vi "Sample-1.vi"() -> ()   [LabVIEW 2016]
uses:
  <vilib>/NI/Modbus Library/API/Modbus API.lvclass/Modbus API.ctl
  <vilib>/NI/Modbus Library/Transmission Data Unit/Transmission Data Unit.lvclass/Transmission Data Unit.ctl
  <vilib>/NI/Modbus Library/Transmission Data Unit/Write Unit ID.vi
  <vilib>/NI/Modbus Library/API/Read Transmission Data Unit.vi
  <vilib>/NI/Modbus Library/API/Write Transmission Data Unit.vi
  <vilib>/NI/Modbus Library/API/Master/Modbus Master.lvclass
  C:/Program Files/National Instruments/LabVIEW 2016/vi.lib/NI/Modbus Library/API/Modbus API.lvclass
  <vilib>/NI/Modbus Library/API/Wrapper/Create TCP Master.vi
  <vilib>/NI/Modbus Library/API/Wrapper/API Main.lvlib
panel:
  in  "stop":bool
  out "Tab Control":T1(tab)
  out "PM-01-FREQ":dbl
  out "PM-01-IAC":dbl
  out "PM-01-VAC":dbl
  out "PM-01-PAC":dbl
  out "SI-01-FREQ":dbl
  out "SI-01-L3":dbl
  out "SI-01-L2":dbl
  out "SI-01-L1":dbl
  out "SI-01-PAC":dbl
  out "SB-02-B-IAC":dbl
  out "SB-02-B-VAC":dbl
  out "SB-02-A-IAC":dbl
  out "SB-02-A-VAC":dbl
  out "SB-02-PAC":dbl
  out "SI-M-FREQ":dbl
  out "SI-M-L3":dbl
  out "SI-M-L2":dbl
  out "SI-M-L1":dbl
  out "SI-M-PAC":dbl
  out "BANK-02-TEMP":dbl
  out "BANK-02-IDC":dbl
  out "BANK-02-VDC":dbl
  out "BANK-02-SOC":dbl
  out "BANK-01-TEMP":dbl
  out "BANK-01-IDC":dbl
  out "BANK-01-VDC":dbl
  out "BANK-01-SOC":dbl
  out "SB-01-B-IAC":dbl
  out "SB-01-B-VAC":dbl
  out "SB-01-A-IAC":dbl
  out "SB-01-A-VAC":dbl
  out "SB-01-PAC":dbl
  in  "Interval":string(combo)
  in  "setting_save_mysql":bool
  in  "db_pwd":string caption="SB-01-IPADDRESS"
  in  "db_username":string caption="SB-01-IPADDRESS"
  in  "db_database":string caption="SB-01-IPADDRESS"
  in  "db_port":string caption="SB-01-IPADDRESS"
  in  "db_host":string caption="SB-01-IPADDRESS"
  in  "db_connection":string caption="SB-01-IPADDRESS"
  in  "setting_save":bool
  in  "SB-04-PORT":string
  in  "SB-04-IPADDRESS":string caption="SB-01-IPADDRESS"
  in  "SB-03-PORT":string
  in  "SB-03-IPADDRESS":string caption="SB-01-IPADDRESS"
  in  "SB-02-PORT":string
  in  "SB-02-IPADDRESS":string caption="SB-01-IPADDRESS"
  in  "SB-01-PORT":string
  in  "SB-01-IPADDRESS":string
  in  "SB-05-IPADDRESS":string caption="SB-01-IPADDRESS"
  in  "SB-05-PORT":string
  in  "Multicolumn Listbox":i32(listbox)
  in  "Path":path
  in  "DATE_END":timestamp format="%<%d/%m/%Y>T"
  in  "DATE_START":timestamp format="%<%d/%m/%Y>T"
  in  "DOWNLOAD":bool
  out "AC_VOLTAGE":cluster{dbl, dbl}[](graph)
  out "BATTERY_CURRENT":cluster{dbl, dbl}[](graph)
  out "SOC":cluster{dbl, dbl}[](graph)
  out "AC_POWER":cluster{dbl, dbl}[](graph)
  in  "Radio Buttons":T2(radio)
  # "RUMAH KUNJAN ( 8.19 kWp )"
  # "SB-01"
  # "BANK-2"
  # "BANK-1"
  # "SB-02"
  # "SOC (%)"
  # "SOC (%)"
  # "Pac (W)"
  # "Pac (W)"
  # "V_bat(V)"
  # "V_bat(V)"
  # "A.Vdc(V)"
  # "A.Vdc(V)"
  # "I_bat(A)"
  # "I_bat(A)"
  # "A.Idc(A)"
  # "A.Idc(A)"
  # "T_bat(°C)"
  # "T_bat(°C)"
  # "B.Vdc(V)"
  # "B.Vdc(V)"
  # "B.Idc(A)"
  # "B.Idc(A)"
  # "SI-M"
  # "SI-01"
  # "Pac (W)"
  # "Pac (W)"
  # "L1"
  # "L1"
  # "L2"
  # "L2"
  # "L3"
  # "L3"
  # "FREQ(HZ)"
  # "FREQ(HZ)"
  # "PM-01"
  # "Pac(W)"
  # "Vac (V)"
  # "Iac(A)"
  # "Freq(Hz)"
  # "SETTING"
  # "MODBUS TCP IP"
  # "MYSQL DATABASE"
  # "SB-01"
  # "DB_CONNECTION :"
  # "IP ADDRESS"
  # "DB_HOST :"
  # "PORT"
  # "DB_PORT  :"
  # "SB-02"
  # "DB_DATABASE  :"
  # "IP ADDRESS"
  # "DB_USERNAME  :"
  # "PORT"
  # "DB_PASSWORD  :"
  # "INTERVAL  :"
  # "SI-M"
  # "IP ADDRESS"
  # "PORT"
  # "SI-01"
  # "IP ADDRESS"
  # "PORT"
  # "DATA MANAGER"
  # "IP ADDRESS"
  # "PORT"
  # "ALERT LIST"
  # "DOWNLOAD DATA"
  # "FILE"
  # "DATE (START)"
  # "DATE (END)"
  # "CHART"
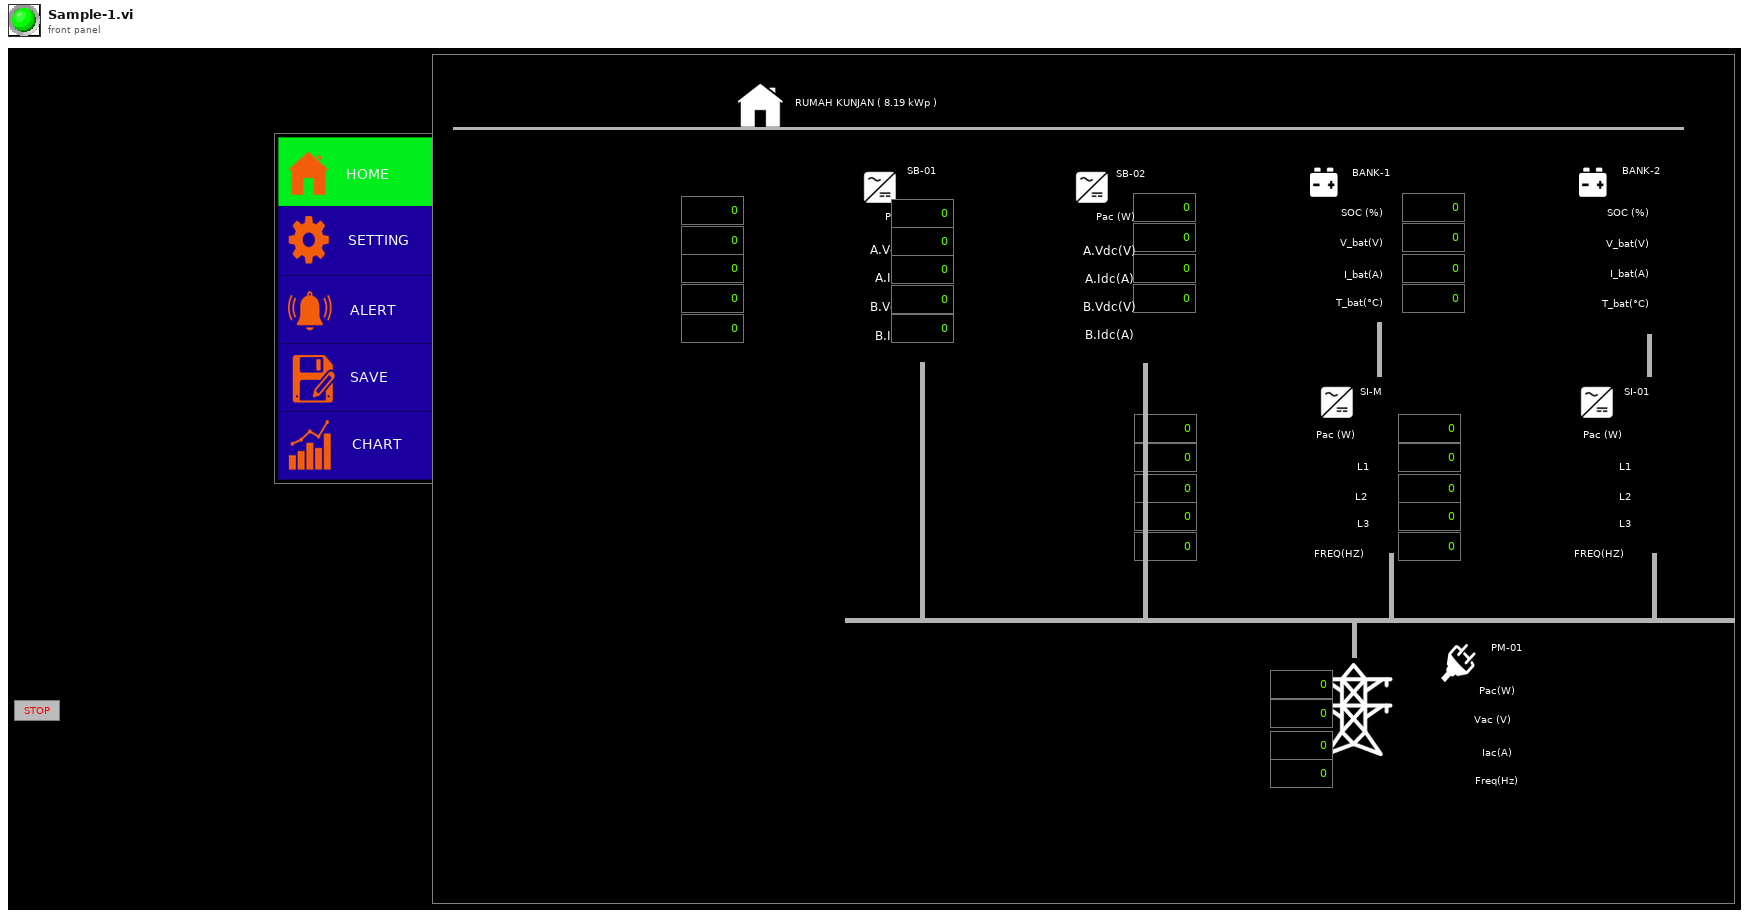
[diagram p1: front panel]
types:
  T1 = enum32{"Page 1", "Page 2", "Page 3", "Page 4", "Page 5"}
  T2 = enum32{"HOME", "SETTING", "ALERT", "SAVE", "CHART"}
  T3 = enum16{"open", "replace", "create", "open or create", "replace or create", "replace or create with confirmation"}
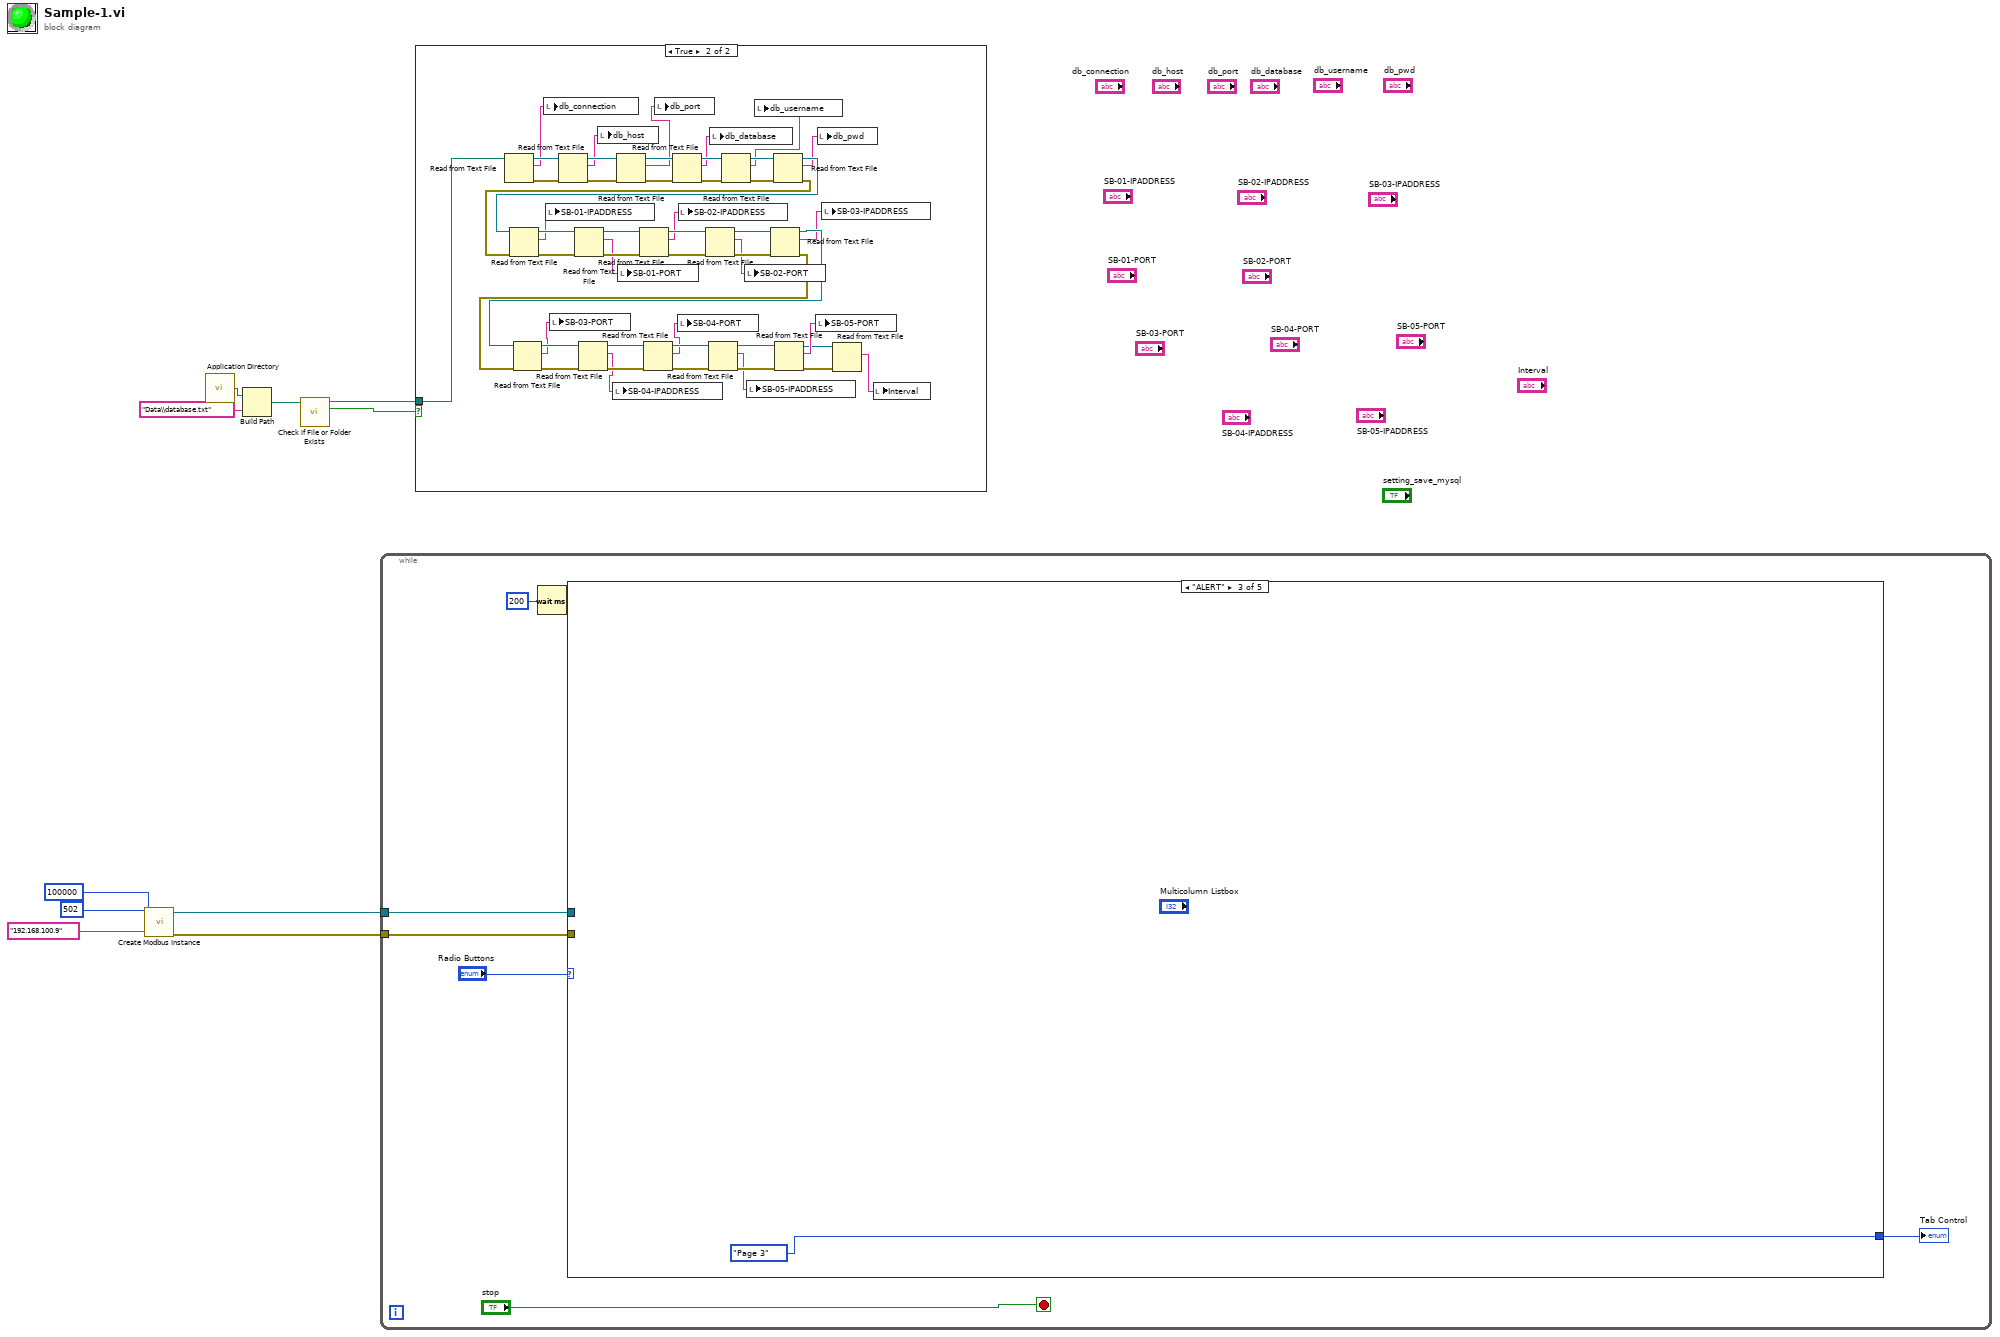
[diagram p0: block diagram]
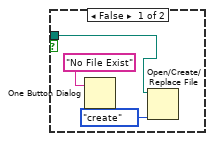
[diagram p2: hidden frame]
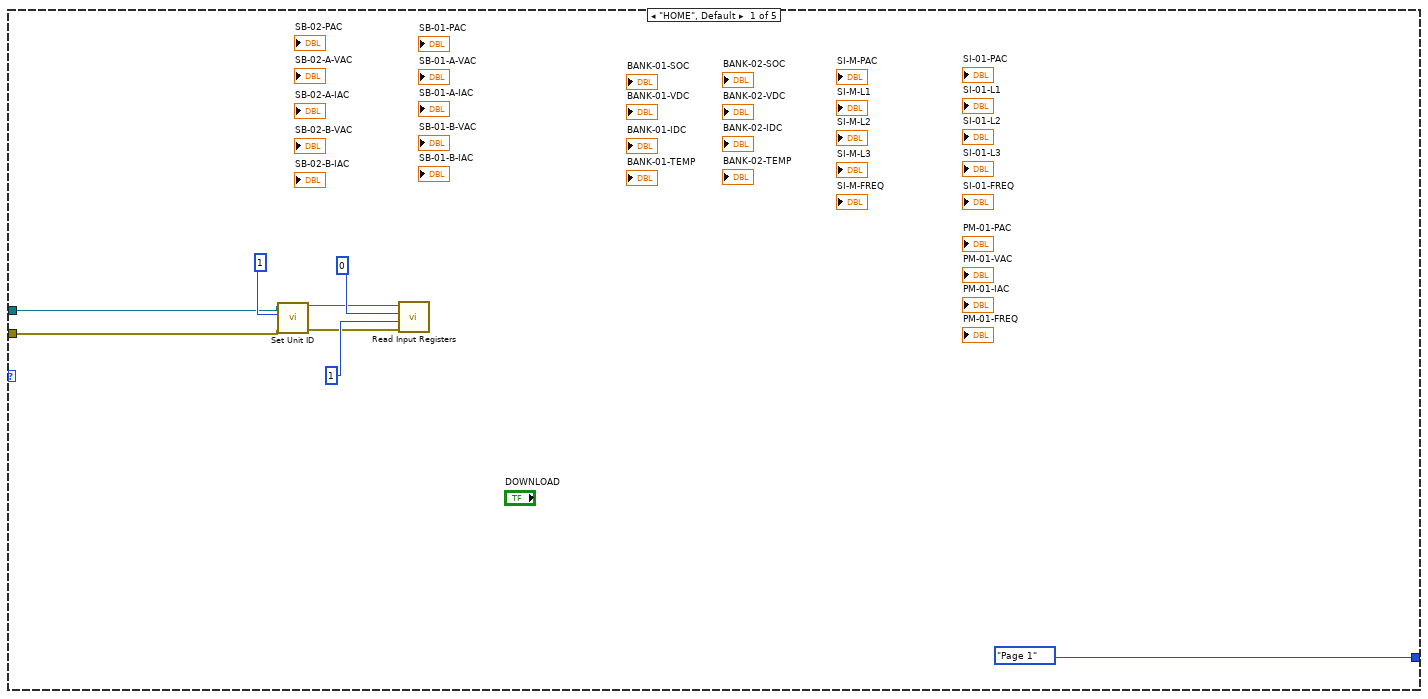
[diagram p3: hidden frame]
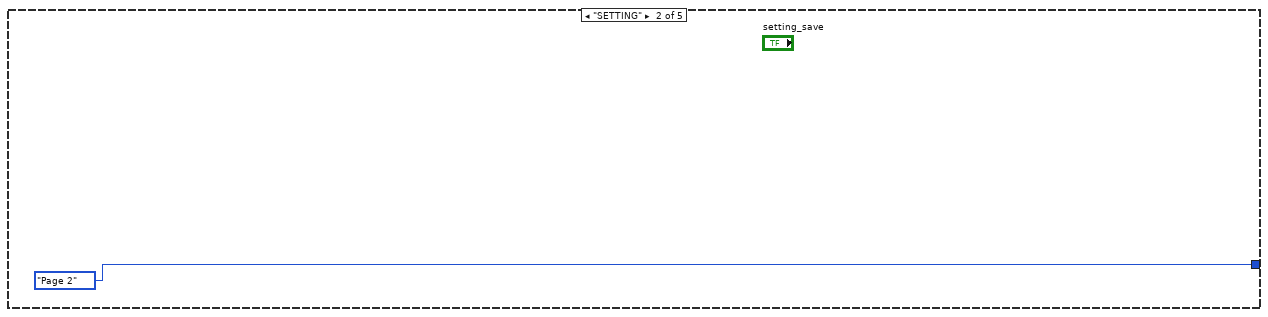
[diagram p4: hidden frame]
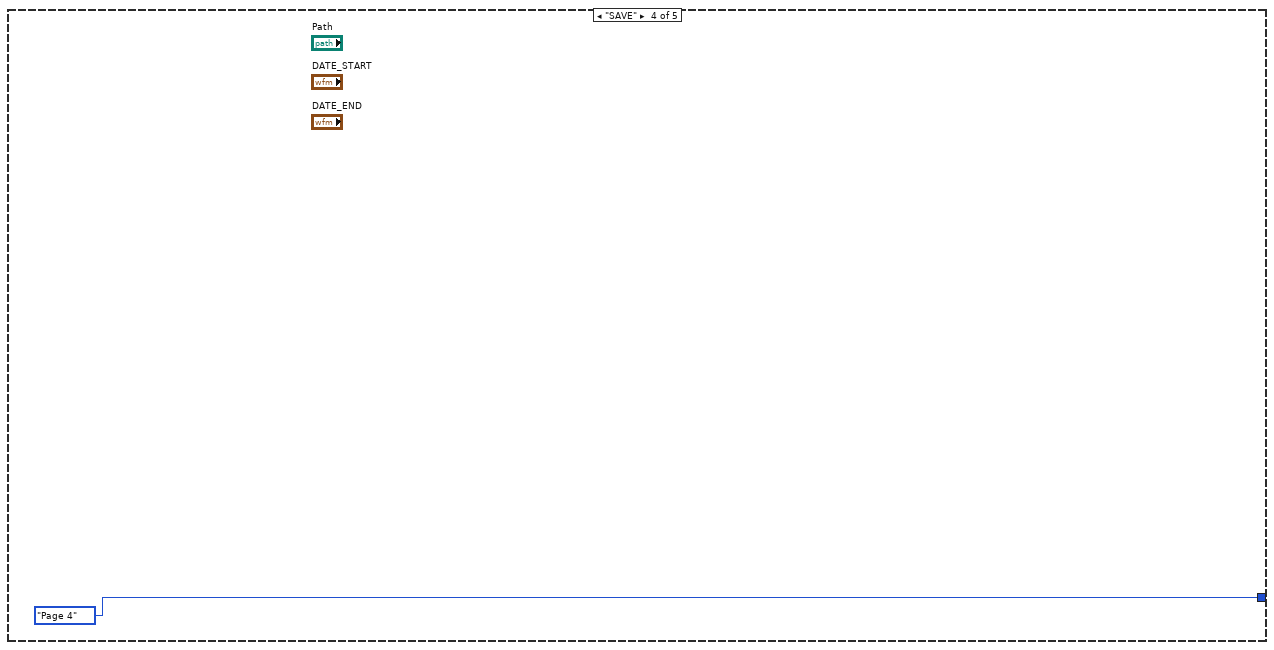
[diagram p5: hidden frame]
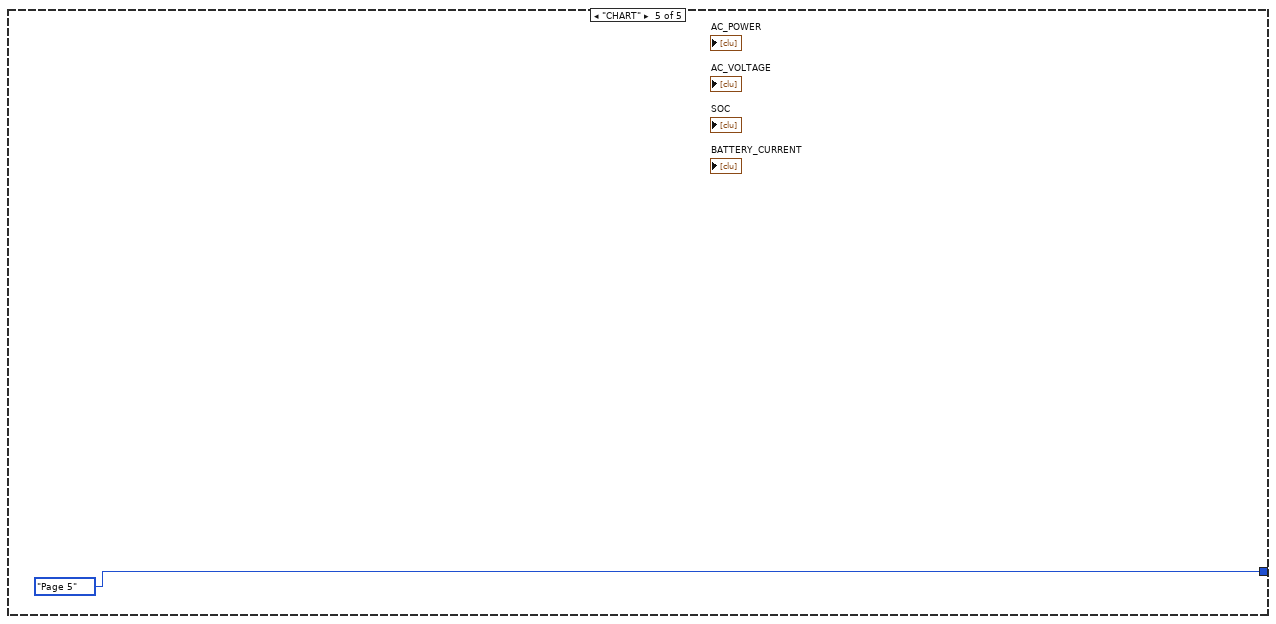
[diagram p6: hidden frame]
diagram:
  n1 = call-poly <vilib>:"Create Modbus Instance.vi"("connect timeout ms"=100000, "port (502)"=u16 502, "address"="192.168.100.9") -> ("error out"=w6:errorcluster, "TCP master instance"=w7:refnum<class "Modbus Master.lvclass">)  [unwired: 7 in]
  n2 = call <vilib>:"Application Directory.vi"() -> ("Application Directory"=w3:path)
  n3 = Build Path(base path=w3, name or relative path="Data\\database.txt") -> (appended path=w5:path)
  n4 = call <vilib>:"Check if File or Folder Exists.vi"("path"=w5) -> ("file or folder exists?"=w1:bool, "dup path"=w2:path)  [unwired: 8 in, 1 out]
  n5 = while {
    tunnel: w7 -> [w14]
    tunnel: w6 -> [w13]
    stop <- "stop" stop-if-true
    n6 = Wait (ms)(milliseconds to wait=u32 200) -> ()  [unwired: 1 out]
    n7 = case shown="\"ALERT\"" "Radio Buttons" {
      tunnel: w14 -> [w19 _ _ _ _]
      tunnel: w13 -> [w18 _ _ _ _]
      tunnel: [T1."Page 1" ("Tab Control") T1."Page 2" ("Tab Control") T1."Page 3" ("Tab Control") T1."Page 4" ("Tab Control") T1."Page 5" ("Tab Control")] -> w11
      frame "HOME", Default {
        n8 = call <vilib>:"Set Unit ID.vi"("error in"=w18, "unit ID"=u8 1, "Modbus master in"=w19) -> ("error out"=w22:errorcluster, "Modbus master out"=w21:refnum<class "Modbus Master.lvclass">)  [unwired: 7 in]
        n9 = call-dynamic "Read Input Registers.vi"("error in"=w22, "number of inputs"=u16 1, "starting address"=u16 0, "Modbus master in"=w21) -> ()  [unwired: 5 in, 3 out]
      }
      frame "SETTING" {
      }
      frame "ALERT" {
      }
      frame "SAVE" {
      }
      frame "CHART" {
      }
    }
    "Tab Control" <- w11
  }
  n10 = case shown="True" w1 {
    tunnel: w2 -> [w30 w81]
    frame False {
      n11 = One Button Dialog(message="No File Exist") -> ()  [unwired: 1 in, 1 out]
      n12 = Open/Create/Replace File(file path (use dialog)=w30, operation (0:open)=T3."create") -> ()  [unwired: 4 in, 3 out]
    }
    frame True {
      n13 = Read from Text File(file (use dialog)=w81) -> (refnum out=w80:refnum<file>, text=w50:string, error out=w76:errorcluster)  [unwired: 3 in, 1 out]
      n14 = local write "db_connection"(w50) -> ()
      n15 = Read from Text File(file (use dialog)=w80, error in=w76) -> (refnum out=w79:refnum<file>, text=w49:string, error out=w75:errorcluster)  [unwired: 2 in, 1 out]
      n16 = local write "db_host"(w49) -> ()
      n17 = Read from Text File(file (use dialog)=w79, error in=w75) -> (refnum out=w78:refnum<file>, text=w48:string, error out=w74:errorcluster)  [unwired: 2 in, 1 out]
      n18 = local write "db_port"(w48) -> ()
      n19 = Read from Text File(file (use dialog)=w78, error in=w74) -> (refnum out=w77:refnum<file>, text=w47:string, error out=w73:errorcluster)  [unwired: 2 in, 1 out]
      n20 = local write "db_database"(w47) -> ()
      n21 = Read from Text File(file (use dialog)=w77, error in=w73) -> (refnum out=w72:refnum<file>, text=w46:string, error out=w71:errorcluster)  [unwired: 2 in, 1 out]
      n22 = local write "db_username"(w46) -> ()
      n23 = Read from Text File(file (use dialog)=w72, error in=w71) -> (refnum out=w69:refnum<file>, text=w45:string, error out=w70:errorcluster)  [unwired: 2 in, 1 out]
      n24 = Read from Text File(file (use dialog)=w69, error in=w70) -> (refnum out=w68:refnum<file>, text=w44:string, error out=w56:errorcluster)  [unwired: 2 in, 1 out]
      n25 = local write "SB-01-IPADDRESS"(w44) -> ()
      n26 = Read from Text File(file (use dialog)=w68, error in=w56) -> (refnum out=w67:refnum<file>, text=w43:string, error out=w55:errorcluster)  [unwired: 2 in, 1 out]
      n27 = local write "SB-01-PORT"(w43) -> ()
      n28 = Read from Text File(file (use dialog)=w67, error in=w55) -> (refnum out=w66:refnum<file>, text=w42:string, error out=w54:errorcluster)  [unwired: 2 in, 1 out]
      n29 = local write "SB-02-IPADDRESS"(w42) -> ()
      n30 = Read from Text File(file (use dialog)=w66, error in=w54) -> (refnum out=w65:refnum<file>, text=w41:string, error out=w53:errorcluster)  [unwired: 2 in, 1 out]
      n31 = local write "SB-02-PORT"(w41) -> ()
      n32 = Read from Text File(file (use dialog)=w65, error in=w53) -> (refnum out=w51:refnum<file>, text=w40:string, error out=w52:errorcluster)  [unwired: 2 in, 1 out]
      n33 = Read from Text File(file (use dialog)=w51, error in=w52) -> (refnum out=w64:refnum<file>, text=w38:string, error out=w60:errorcluster)  [unwired: 2 in, 1 out]
      n34 = local write "SB-03-PORT"(w38) -> ()
      n35 = Read from Text File(file (use dialog)=w64, error in=w60) -> (refnum out=w63:refnum<file>, text=w39:string, error out=w59:errorcluster)  [unwired: 2 in, 1 out]
      n36 = local write "SB-04-IPADDRESS"(w39) -> ()
      n37 = Read from Text File(file (use dialog)=w63, error in=w59) -> (refnum out=w62:refnum<file>, text=w37:string, error out=w58:errorcluster)  [unwired: 2 in, 1 out]
      n38 = local write "SB-04-PORT"(w37) -> ()
      n39 = Read from Text File(file (use dialog)=w62, error in=w58) -> (refnum out=w61:refnum<file>, text=w36:string, error out=w57:errorcluster)  [unwired: 2 in, 1 out]
      n40 = local write "SB-05-IPADDRESS"(w36) -> ()
      n41 = Read from Text File(file (use dialog)=w61, error in=w57) -> (refnum out=w34:refnum<file>, text=w35:string, error out=w33:errorcluster)  [unwired: 2 in, 1 out]
      n42 = local write "SB-05-PORT"(w35) -> ()
      n43 = local write "db_pwd"(w45) -> ()
      n44 = local write "SB-03-IPADDRESS"(w40) -> ()
      n45 = Read from Text File(file (use dialog)=w34, error in=w33) -> (text=w32:string)  [unwired: 2 in, 3 out]
      n46 = local write "Interval"(w32) -> ()
    }
  }
